vi "fault and error bookkeeping.vi"(0 "data table in":T9, 1 "worker pool reference":T2, 5 "module data":T5={"run state"=enum."sync", "module"=refnum, "module ref"=refnum, "async exec ref"={"command fifo"=refnum, "error fifo"=refnum, "input buffer"=refnum, "output buffer"=refnum, "process buffer"=refnum, "original dvrs"=[]}, "configuration ref"=refnum, "error"={"status"=FALSE, "code"=0, "source"=""}, "previous error code"=0, "input method"={"data table"={"Double"=[], "Single"=[], "I64"=[], "I32"=[], "I16"=[], "I8"=[], "U64"=[], "U32"=[], "U16"=[], "U8"=[], "Boolean"=[], "String"=[], "Array of Double"=[], "Array of Single"=[], "Array of I64"=[], "Array of I32"=[], "Array of I16"=[], "Array of I8"=[], "Array of U64"=[], "Array of U32"=[], "Array of U16"=[], "Array of U8"=[], "Array of Boolean"=[], "Array of String"=[]}, "transfer spec"=[]}, "output method"={"data table"={"Double"=[], "Single"=[], "I64"=[], "I32"=[], "I16"=[], "I8"=[], "U64"=[], "U32"=[], "U16"=[], "U8"=[], "Boolean"=[], "String"=[], "Array of Double"=[], "Array of Single"=[], "Array of I64"=[], "Array of I32"=[], "Array of I16"=[], "Array of I8"=[], "Array of U64"=[], "Array of U32"=[], "Array of U16"=[], "Array of U8"=[], "Array of Boolean"=[], "Array of String"=[]}, "transfer spec"=[]}, "process method parameters"={"data table"={"Double"=[], "Single"=[], "I64"=[], "I32"=[], "I16"=[], "I8"=[], "U64"=[], "U32"=[], "U16"=[], "U8"=[], "Boolean"=[], "String"=[], "Array of Double"=[], "Array of Single"=[], "Array of I64"=[], "Array of I32"=[], "Array of I16"=[], "Array of I8"=[], "Array of U64"=[], "Array of U32"=[], "Array of U16"=[], "Array of U8"=[], "Array of Boolean"=[], "Array of String"=[]}, "transfer spec"=[]}, "process method results"={"data table"={"Double"=[], "Single"=[], "I64"=[], "I32"=[], "I16"=[], "I8"=[], "U64"=[], "U32"=[], "U16"=[], "U8"=[], "Boolean"=[], "String"=[], "Array of Double"=[], "Array of Single"=[], "Array of I64"=[], "Array of I32"=[], "Array of I16"=[], "Array of I8"=[], "Array of U64"=[], "Array of U32"=[], "Array of U16"=[], "Array of U8"=[], "Array of Boolean"=[], "Array of String"=[]}, "transfer spec"=[]}, "fault handling"={"unknown"=[], "trivial"=[], "critical"=[], "recoverable"=[]}, "error report index "=-1}, 7 "time data in":T1, 9 "run flags in":u8, 11 "engine error in":errorcluster, 12 "module index":i32) -> (4 "data table out":T9, 6 "module data out":T5={"run state"=enum."sync", "module"=refnum, "module ref"=refnum, "async exec ref"={"command fifo"=refnum, "error fifo"=refnum, "input buffer"=refnum, "output buffer"=refnum, "process buffer"=refnum, "original dvrs"=[]}, "configuration ref"=refnum, "error"={"status"=FALSE, "code"=0, "source"=""}, "previous error code"=0, "input method"={"data table"={"Double"=[], "Single"=[], "I64"=[], "I32"=[], "I16"=[], "I8"=[], "U64"=[], "U32"=[], "U16"=[], "U8"=[], "Boolean"=[], "String"=[], "Array of Double"=[], "Array of Single"=[], "Array of I64"=[], "Array of I32"=[], "Array of I16"=[], "Array of I8"=[], "Array of U64"=[], "Array of U32"=[], "Array of U16"=[], "Array of U8"=[], "Array of Boolean"=[], "Array of String"=[]}, "transfer spec"=[]}, "output method"={"data table"={"Double"=[], "Single"=[], "I64"=[], "I32"=[], "I16"=[], "I8"=[], "U64"=[], "U32"=[], "U16"=[], "U8"=[], "Boolean"=[], "String"=[], "Array of Double"=[], "Array of Single"=[], "Array of I64"=[], "Array of I32"=[], "Array of I16"=[], "Array of I8"=[], "Array of U64"=[], "Array of U32"=[], "Array of U16"=[], "Array of U8"=[], "Array of Boolean"=[], "Array of String"=[]}, "transfer spec"=[]}, "process method parameters"={"data table"={"Double"=[], "Single"=[], "I64"=[], "I32"=[], "I16"=[], "I8"=[], "U64"=[], "U32"=[], "U16"=[], "U8"=[], "Boolean"=[], "String"=[], "Array of Double"=[], "Array of Single"=[], "Array of I64"=[], "Array of I32"=[], "Array of I16"=[], "Array of I8"=[], "Array of U64"=[], "Array of U32"=[], "Array of U16"=[], "Array of U8"=[], "Array of Boolean"=[], "Array of String"=[]}, "transfer spec"=[]}, "process method results"={"data table"={"Double"=[], "Single"=[], "I64"=[], "I32"=[], "I16"=[], "I8"=[], "U64"=[], "U32"=[], "U16"=[], "U8"=[], "Boolean"=[], "String"=[], "Array of Double"=[], "Array of Single"=[], "Array of I64"=[], "Array of I32"=[], "Array of I16"=[], "Array of I8"=[], "Array of U64"=[], "Array of U32"=[], "Array of U16"=[], "Array of U8"=[], "Array of Boolean"=[], "Array of String"=[]}, "transfer spec"=[]}, "fault handling"={"unknown"=[], "trivial"=[], "critical"=[], "recoverable"=[]}, "error report index "=-1}, 8 "safe state?":bool, 10 "run flags out":u8, 15 "engine error out":errorcluster)   [LabVIEW 2013, in "main engine.lvlib"]
doc: "Performs error handling actions for modules running both synchronously and asynchronously."
uses:
  main engine.lvlib
  <vilib>/NI/Tag Bus/table/data table.ctl
  full module data.ctl
  <vilib>/NI/Tag Bus Module Framework/runtime/TBM module execution interface.lvclass
  module run state.ctl
  async executor/asynchronous executor reference.ctl
  async executor/async message to executor.ctl
  Runtime/async command notification.ctl
  Runtime/async error info.ctl
  <vilib>/NI/Tag Bus Module Framework/runtime/error classification.ctl
  <vilib>/NI/Tag Bus Module Framework/module configuration/TBM module configuration.lvclass
  module method data.ctl
  <vilib>/NI/Tag Bus/table/transfer specification.ctl
  <vilib>/NI/Tag Bus/tag/Data Type.ctl
  fault handling spec.ctl
  Configuration/Error Actions.ctl
  worker library/worker comms.ctl
  worker library/worker commands.ctl
  worker library/request fifos.ctl
  worker library/recovery request.ctl
  worker library/rt fault.ctl
  worker library/response fifos.ctl
  worker library/recovery response.ctl
  <vilib>/NI/Module Execution Interface/Engine Runtime/Fault.ctl
  time information.ctl
  <vilib>/NI/Tag Bus/table/data polymorphs/write one/write I32.vi
  <vilib>/NI/Tag Bus/table/data table.lvlib
  worker library/worker pool.lvlib
  Configuration/Standard Engine Configuration.lvclass
  <vilib>/NI/Tag Bus/tag/tag descriptor.lvclass
  <vilib>/NI/Module Execution Interface/Engine Runtime/Engine Runtime Interface.lvclass
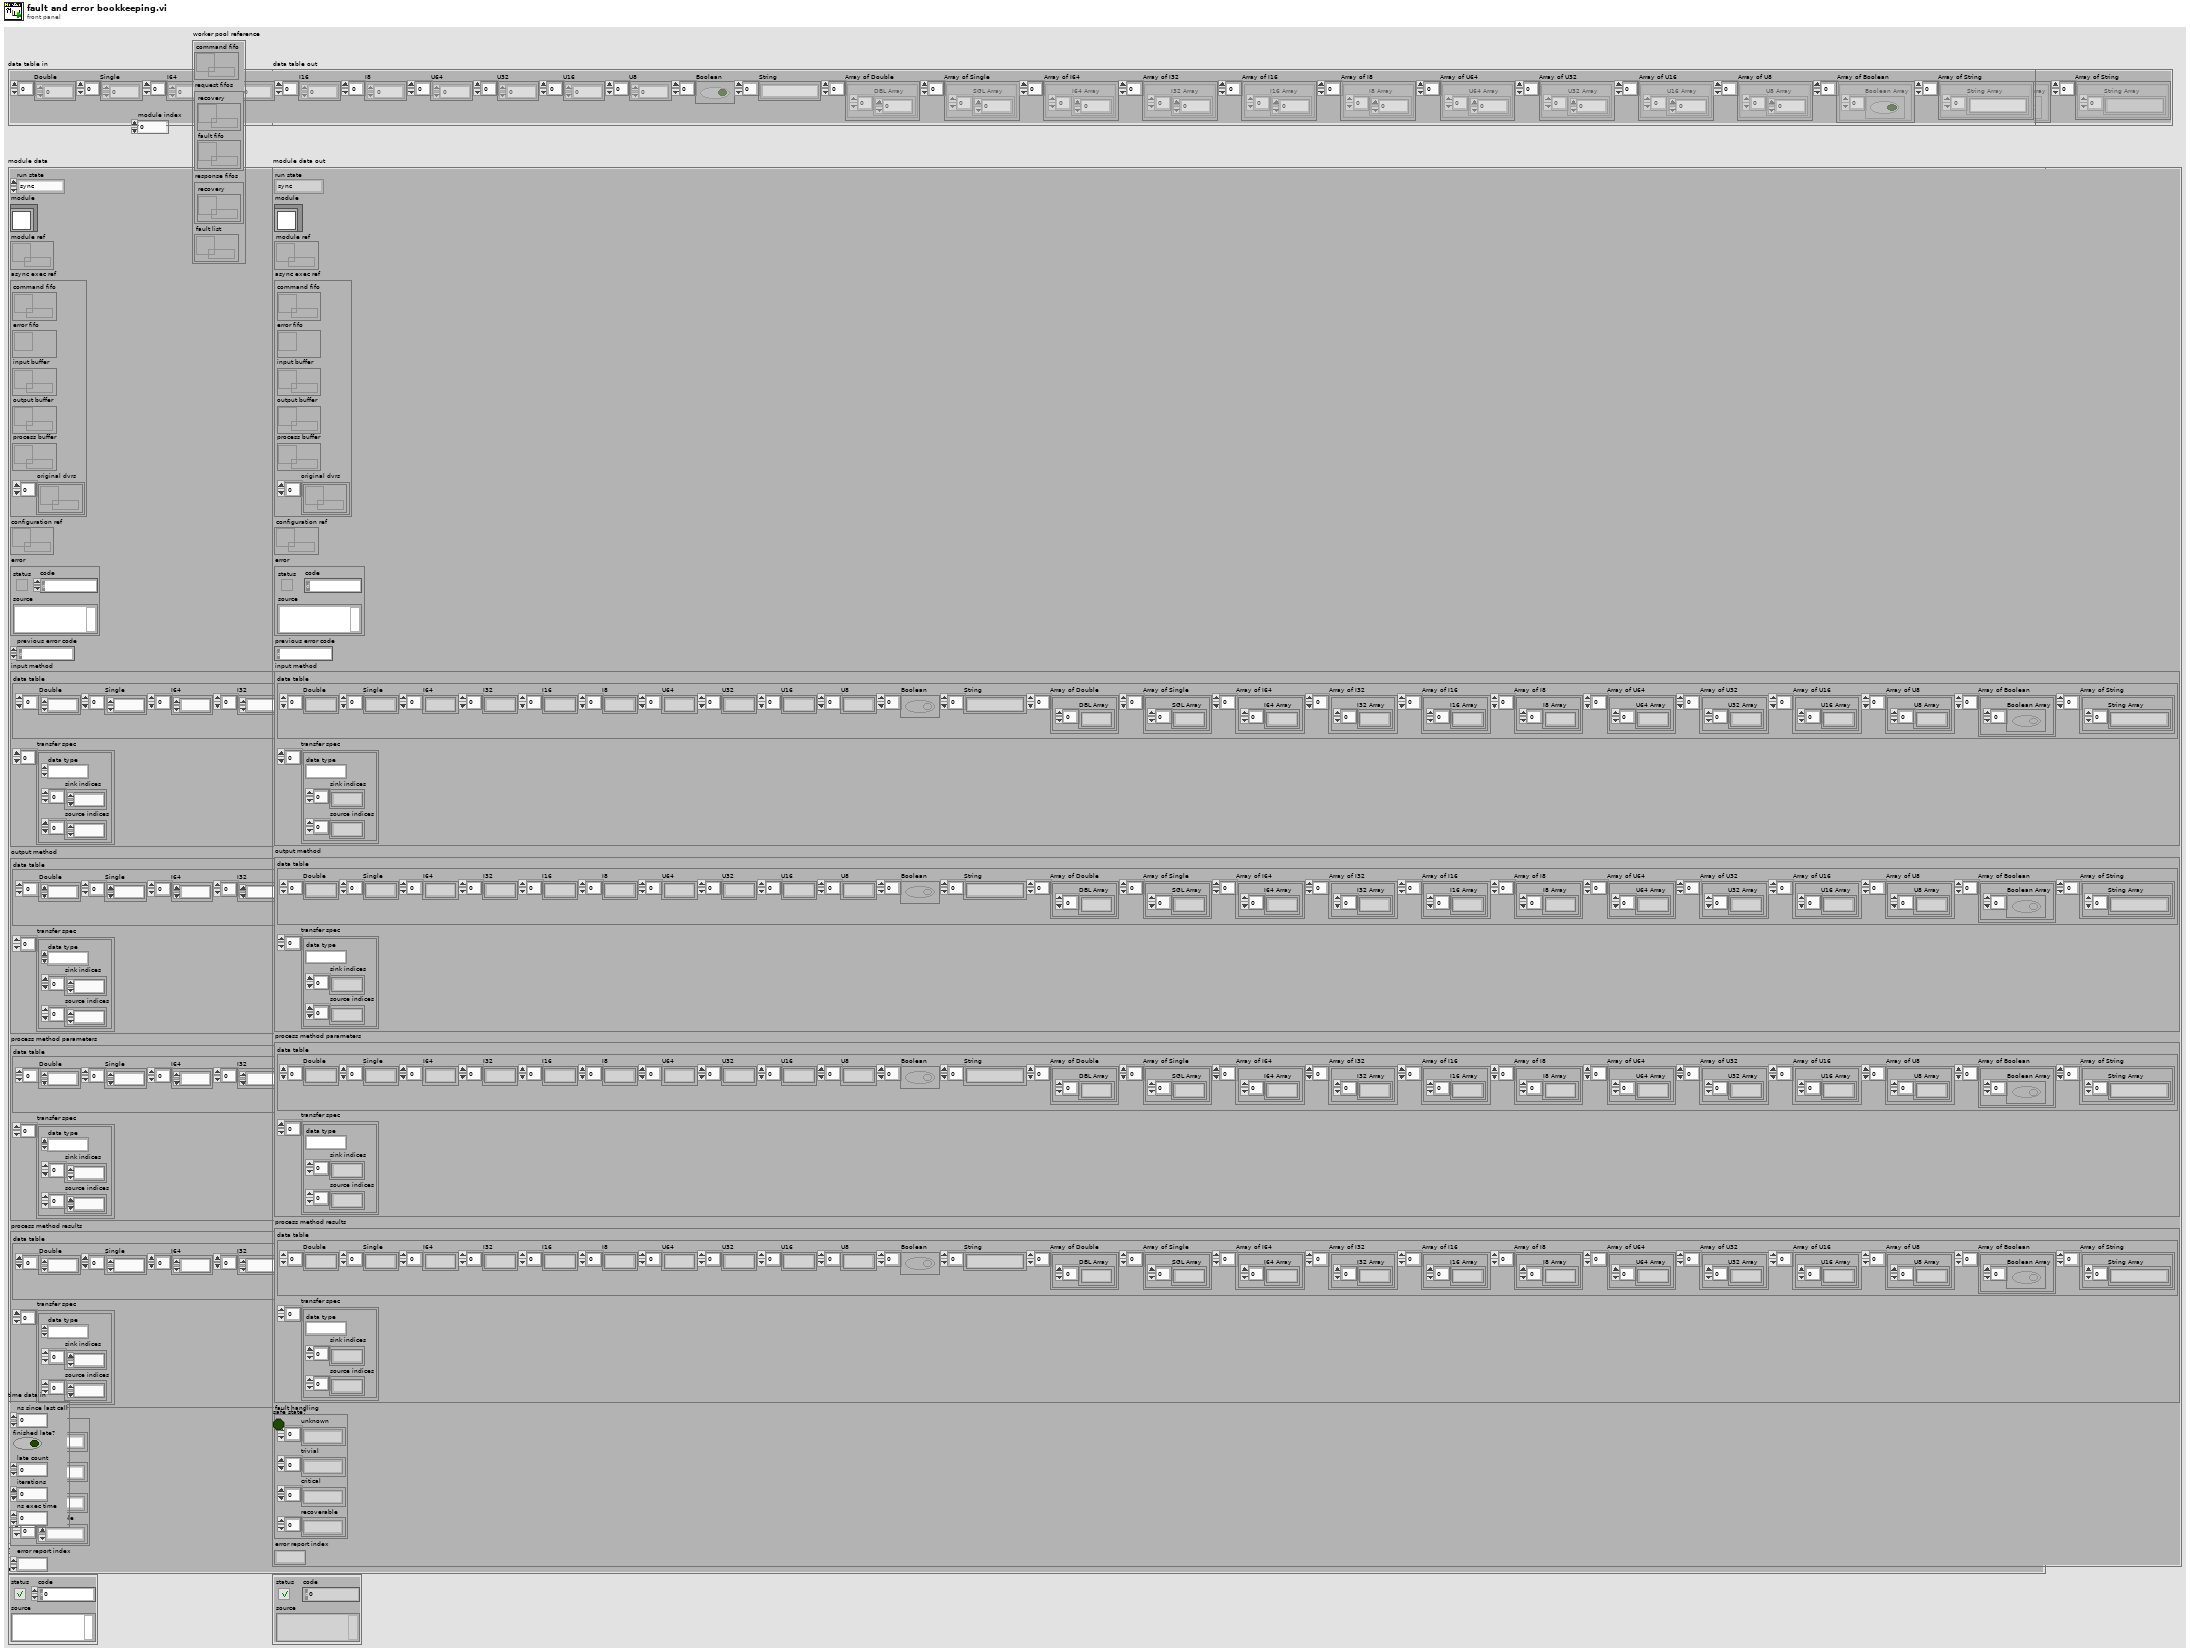
[diagram p1: front panel]
types:
  T1 = typedef "main engine.lvlib/time information.ctl" = cluster{"ns since last call":u64, "finished late?":bool, "late count":u32, "iterations":u64, "ns exec time":u64}
  T2 = typedef "worker pool.lvlib/worker comms.ctl" = cluster{"command fifo":refnum<k33>, "request fifos":T3, "response fifos":T4, "fault list":refnum<data-value>}
  T3 = typedef "worker pool.lvlib/request fifos.ctl" = cluster{"recovery":refnum<k33>, "fault fifo":refnum<k33>}
  T4 = typedef "worker pool.lvlib/response fifos.ctl" = cluster{"recovery":refnum<k33>}
  T5 = typedef "main engine.lvlib/full module data.ctl" = cluster{"run state":T6, "module":refnum<class "TBM module execution interface.lvclass">, "module ref":refnum<data-value>, "async exec ref":T7, "configuration ref":refnum<data-value>, "error":errorcluster, "previous error code":i32, "input method":T8, "output method":T8, "process method parameters":T8, "process method results":T8, "fault handling":T12, "error report index ":i32}
  T6 = typedef "main engine.lvlib/module run state.ctl" = enum16{"sync", "async"}
  T7 = typedef "main engine.lvlib/asynchronous executor reference.ctl" = cluster{"command fifo":refnum<k33>, "error fifo":refnum<k33>, "input buffer":refnum<k33>, "output buffer":refnum<k33>, "process buffer":refnum<k33>, "original dvrs":refnum<data-value>[]}
  T8 = typedef "main engine.lvlib/module method data.ctl" = cluster{"data table":T9, "transfer spec":T10[]}
  T9 = typedef "tag bus.lvlib/data table.lvlib/data table.ctl" = cluster{"Double":dbl[], "Single":sgl[], "I64":i64[], "I32":i32[], "I16":i16[], "I8":i8[], "U64":u64[], "U32":u32[], "U16":u16[], "U8":u8[], "Boolean":bool[], "String":string[], "Array of Double":cluster{"DBL Array":dbl[]}[], "Array of Single":cluster{"SGL Array":sgl[]}[], "Array of I64":cluster{"I64 Array":i64[]}[], "Array of I32":cluster{"I32 Array":i32[]}[], "Array of I16":cluster{"I16 Array":i16[]}[], "Array of I8":cluster{"I8 Array":i8[]}[], "Array of U64":cluster{"U64 Array":u64[]}[], "Array of U32":cluster{"U32 Array":u32[]}[], "Array of U16":cluster{"U16 Array":u16[]}[], "Array of U8":cluster{"U8 Array":u8[]}[], "Array of Boolean":cluster{"Boolean Array":bool[]}[], "Array of String":cluster{"String Array":string[]}[]}
  T10 = typedef "tag bus.lvlib/data table.lvlib/transfer specification.ctl" = cluster{"data type":T11, "sink indices":i32[], "source indices":i32[]}
  T11 = typedef "tag bus.lvlib/tag descriptor.lvclass/Data Type.ctl" = enum16{"Double", "Single", "I64", "I32", "I16", "I8", "U64", "U32", "U16", "U8", "Boolean", "String", "Array of Double", "Array of Single", "Array of I64", "Array of I32", "Array of I16", "Array of I8", "Array of U64", "Array of U32", "Array of U16", "Array of U8", "Array of Boolean", "Array of String"}
  T12 = typedef "main engine.lvlib/fault handling spec.ctl" = cluster{"unknown":T13[], "trivial":T13[], "critical":T13[], "recoverable":T13[]}
  T13 = typedef "Standard Engine Configuration.lvclass/Error Actions.ctl" = enum16{"Clear", "Notify", "Log", "Stop Component", "Stop Engine", "Safe State", "Attempt Recovery"}
  T14 = typedef "TBM module execution interface.lvclass/error classification.ctl" = enum16{"unknown", "none", "trivial", "recoverable", "critical"}
  T15 = typedef "main engine.lvlib/async error info.ctl" = cluster{"error code":i32, "error classification":T14}
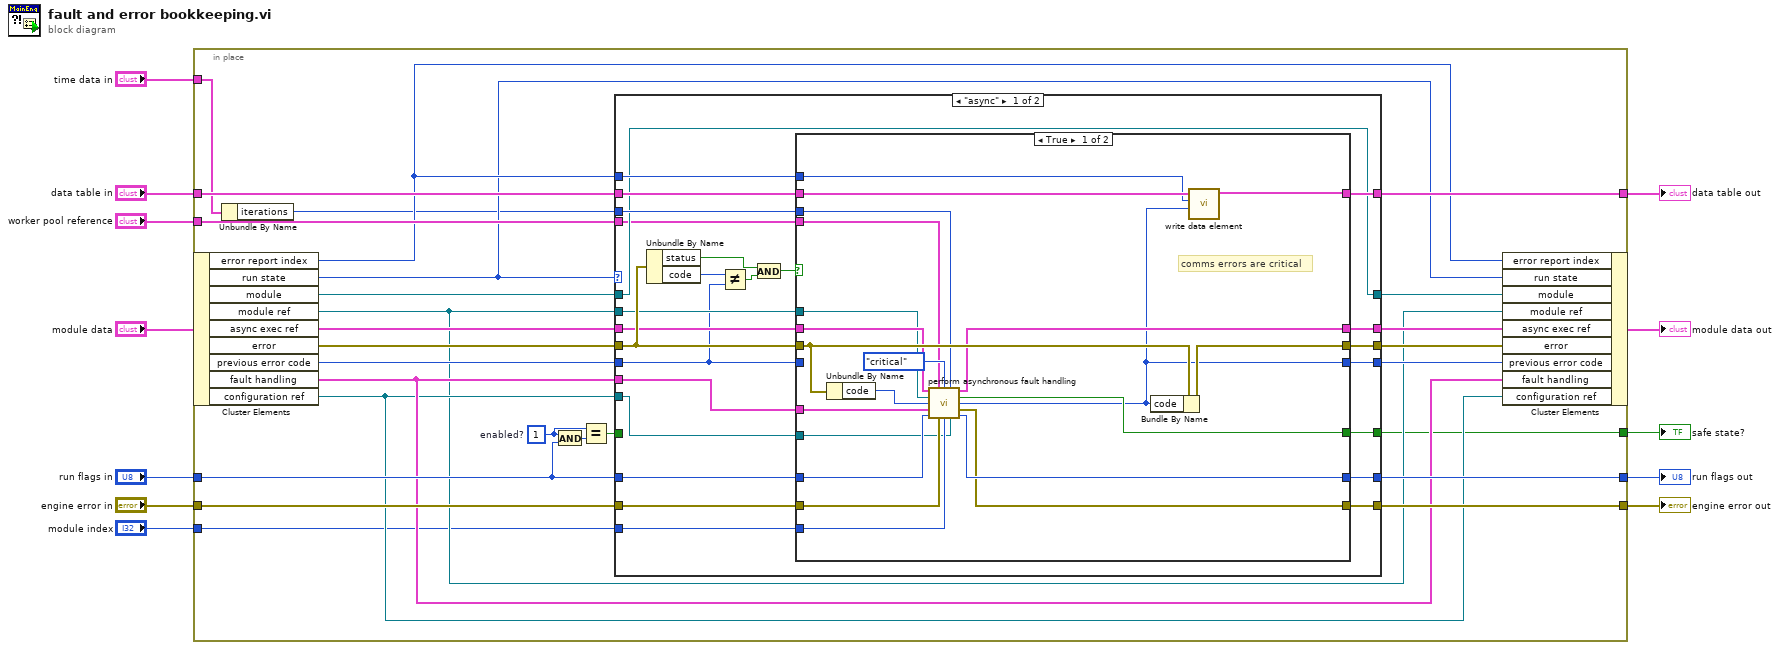
[diagram p0: block diagram]
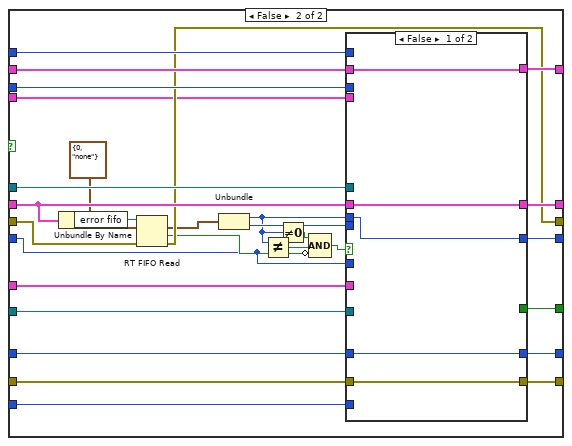
[diagram p2: hidden frame]
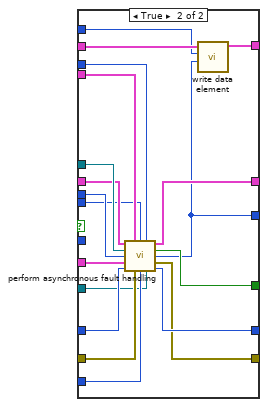
[diagram p3: hidden frame]
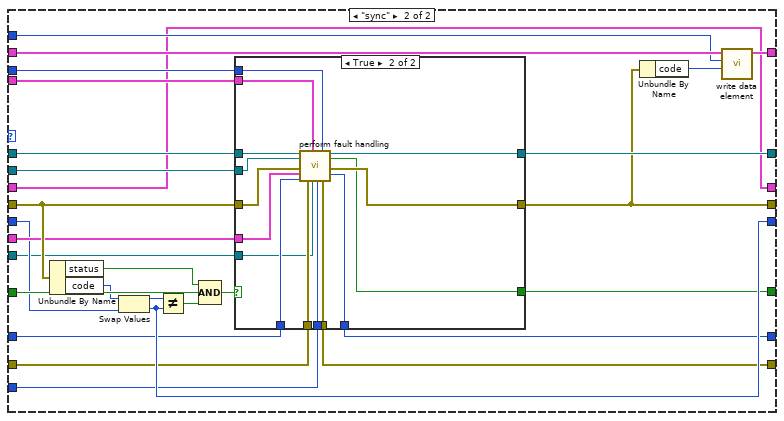
[diagram p4: hidden frame]
diagram:
  n1 = in-place {
    in-place-border: [w39] -> w12
    in-place-border: "run flags in" -> [w38]
    in-place-border: [w34] -> w10
    in-place-border: "data table in" -> [w33]
    in-place-border: "engine error in" -> [w32]
    in-place-border: [w31] -> w7
    in-place-border: "worker pool reference" -> [w30]
    in-place-border: "time data in" -> [w16]
    in-place-border: "module index" -> [w15]
    in-place-border: [w13] -> w1
    w36 = u8 1  # enabled?
    n2 = in-place-cluster #1("module data") -> ("error report index"=w29:i32, "run state"=w28:T6, "module"=w27:refnum<class "TBM module execution interface.lvclass">, "module ref"=w17:refnum<data-value>, "async exec ref"=w26:T7, "error"=w25:errorcluster, "previous error code"=w24:i32, "fault handling"=w19:T12, "configuration ref"=w18:refnum<data-value>)
    n3 = Unbundle By Name(w16) -> ("iterations"=w14:u64)
    n4 = And(x=w36, y=w38) -> (x .and. y?=w35:u8)
    n5 = Equal?(x=w36, y=w35) -> (x = y?=w37:bool)
    n6 = case shown="\"async\"" w28 {
      tunnel: w33 -> [w63 w166]
      tunnel: [w62 w165] -> w34
      tunnel: w29 -> [w61 w164]
      tunnel: w37 -> [_ w163]
      tunnel: w27 -> [w41 w161]
      tunnel: [w41 w160] -> w20
      tunnel: [w57 w139] -> w21
      tunnel: w26 -> [w58 w139]
      tunnel: w25 -> [w59 w159]
      tunnel: w19 -> [w46 w158]
      tunnel: [w60 w149] -> w22
      tunnel: w17 -> [w49 w156]
      tunnel: w24 -> [w42 w152]
      tunnel: [w56 w151] -> w23
      tunnel: [w55 w147] -> w39
      tunnel: w38 -> [w54 w148]
      tunnel: w32 -> [w53 w146]
      tunnel: [w48 w145] -> w31
      tunnel: w30 -> [w40 w142]
      tunnel: w18 -> [w47 w144]
      tunnel: w15 -> [w52 w143]
      tunnel: w14 -> [w50 w141]
      tunnel: [w51 w140] -> w13
      frame "async" {
        n7 = Unbundle By Name(w59) -> ("status"=w64:bool, "code"=w43:i32)
        n8 = Not Equal?(x=w43, y=w42) -> (x != y?=w44:bool)
        n9 = And(x=w64, y=w44) -> (x .and. y?=w45:bool)
        n10 = case shown="True" w45 {
          tunnel: w63 -> [w84 w113]
          tunnel: [w85 w114] -> w62
          tunnel: w61 -> [w83 w112]
          tunnel: [w72 w97] -> w60
          tunnel: w59 -> [w82 w111]
          tunnel: w58 -> [w75 w98]
          tunnel: [w76 w105] -> w57
          tunnel: [w67 w99] -> w56
          tunnel: [w79 w108] -> w55
          tunnel: w54 -> [w78 w107]
          tunnel: w53 -> [w81 w110]
          tunnel: w52 -> [w80 w109]
          tunnel: [w77 w106] -> w51
          tunnel: w50 -> [w74 w104]
          tunnel: w49 -> [w71 w103]
          tunnel: [w70 w102] -> w48
          tunnel: w47 -> [w69 w101]
          tunnel: w46 -> [w68 w100]
          tunnel: w42 -> [_ w92]
          tunnel: w40 -> [w65 w86]
          frame True {
            # "comms errors are critical"
            n11 = Unbundle By Name(w82) -> ("code"=w73:i32)
            n12 = call "perform asynchronous fault handling.vi"("module in"=w75, "worker pool reference"=w65, "error classification"=error_classification."critical", "iteration"=w74, "module ref in"=w71, "code"=w73, "fault handling in"=w68, "run flags in"=w78, "engine error in"=w81, "engine reference"=w80, "cfg ref"=w69) -> ("module out"=w76:T7, "go to safe state"=w77:bool, "code out"=w67:i32, "engine error out"=w70:errorcluster, "run flags out"=w79:u8)
            n13 = Bundle By Name(cluster=w82, "code"=w67) -> (w72:errorcluster)
            n14 = call-poly <vilib>:"write data element.vi"("value"=w67, "index"=w83, "data table in"=w84) -> ("data table out"=w85:T9)  [unwired: 8 in]
          }
          frame False {
            n15 = Unbundle By Name(w98) -> ("error fifo"=w96:refnum<k33>)
            n16 = RT FIFO Read(0:w96, 1:T15 {"error code"=0, "error classification"=enum."none"} ("element"), 3:w111) -> (9:w93:T15, 10:w95:bool, 11:w97:errorcluster)  [unwired: 1 in, 2 out]
            n17 = Unbundle(w93) -> ("error code"=w87:i32, "error classification"=w90:T14)
            n18 = Not Equal?(x=w87, y=w92) -> (x != y?=w91:bool)
            n19 = Not Equal To 0?(x=w87) -> (x != 0?=w88:bool)
            n20 = Compound Arithmetic op=AND(w88, w91, invert w95) -> (w94:bool)
            n21 = case shown="False" w94 {
              tunnel: [w119 w138] -> w114
              tunnel: w113 -> [w119 w137]
              tunnel: w112 -> [_ w136]
              tunnel: w110 -> [w116 w135]
              tunnel: w109 -> [_ w134]
              tunnel: [w117 w133] -> w108
              tunnel: w107 -> [w117 w132]
              tunnel: [_ w131] -> w106
              tunnel: [w118 w130] -> w105
              tunnel: w86 -> [_ w129]
              tunnel: w104 -> [_ w128]
              tunnel: w103 -> [_ w127]
              tunnel: [w116 w126] -> w102
              tunnel: w101 -> [_ w125]
              tunnel: w100 -> [_ w124]
              tunnel: [w115 w123] -> w99
              tunnel: w98 -> [w118 w122]
              tunnel: w92 -> [_ _]
              tunnel: w87 -> [w115 w121]
              tunnel: w90 -> [_ w120]
              frame False {
              }
              frame True {
                n22 = call "perform asynchronous fault handling.vi"("module in"=w122, "worker pool reference"=w129, "error classification"=w120, "iteration"=w128, "module ref in"=w127, "code"=w121, "fault handling in"=w124, "run flags in"=w132, "engine error in"=w135, "engine reference"=w134, "cfg ref"=w125) -> ("module out"=w130:T7, "go to safe state"=w131:bool, "code out"=w123:i32, "engine error out"=w126:errorcluster, "run flags out"=w133:u8)
                n23 = call-poly <vilib>:"write data element.vi"("value"=w123, "index"=w136, "data table in"=w137) -> ("data table out"=w138:T9)  [unwired: 8 in]
              }
            }
          }
        }
      }
      frame "sync" {
        n24 = Unbundle By Name(w159) -> ("status"=w157:bool, "code"=w153:i32)
        n25 = Swap Values(12:w153, 14:w152) -> (1:w154:i32, 3:w151:i32)  [unwired: 1 in]
        n26 = Not Equal?(x=w154, y=w151) -> (x != y?=w155:bool)
        n27 = Compound Arithmetic op=AND(w157, w163, w155) -> (w162:bool)
        n28 = case shown="True" w162 {
          tunnel: w161 -> [w170 w184]
          tunnel: [w170 w185] -> w160
          tunnel: w159 -> [w169 w180]
          tunnel: [w169 w182] -> w149
          tunnel: w158 -> [_ w181]
          tunnel: w156 -> [_ w183]
          tunnel: w148 -> [w168 w179]
          tunnel: [w168 w178] -> w147
          tunnel: w146 -> [w167 w177]
          tunnel: [w167 w176] -> w145
          tunnel: w144 -> [_ w175]
          tunnel: w143 -> [_ w174]
          tunnel: w142 -> [_ w173]
          tunnel: w141 -> [_ w172]
          tunnel: [_ w171] -> w140
          frame False {
          }
          frame True {
            n29 = call "perform fault handling.vi"("module in"=w184, "module ref in"=w183, "error in"=w180, "fault handling in"=w181, "run flags in"=w179, "engine error in"=w177, "worker pool in"=w173, "cfg ref"=w175, "engine reference"=w174, "iteration"=w172) -> ("engine error out"=w176:errorcluster, "module out"=w185:refnum<class "TBM module execution interface.lvclass">, "go to safe state"=w171:bool, "error out"=w182:errorcluster, "run flags out"=w178:u8)  [unwired: 5 in]
          }
        }
        n30 = Unbundle By Name(w149) -> ("code"=w150:i32)
        n31 = call-poly <vilib>:"write data element.vi"("value"=w150, "index"=w164, "data table in"=w166) -> ("data table out"=w165:T9)  [unwired: 8 in]
      }
    }
    n32 = in-place-cluster #1("error report index"=w29, "run state"=w28, "module"=w20, "module ref"=w17, "async exec ref"=w21, "error"=w22, "previous error code"=w23, "fault handling"=w19, "configuration ref"=w18) -> (→"module data out":T5)
  }
  "run flags out" <- w12
  "data table out" <- w10
  "engine error out" <- w7
  "safe state?" <- w1
